vi "vipm_OpenVIPM.vi"(8 "error in (no error)":errorcluster, 11 "CommandLine":string[](array[string])) -> (0 "error out":errorcluster, 2 "test details":string, 3 "output to action":string)   [LabVIEW 2014]
uses:
  _lvcicd/_lvcicd_support_2014.lvlib
  <vilib>/JKI/VIPM API/VIPM API_vipm_api.lvlib
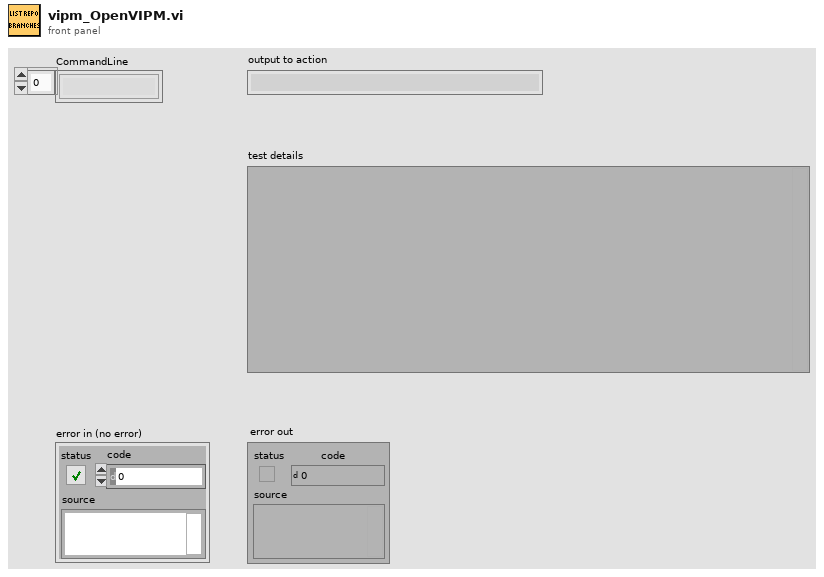
[diagram p1: front panel]
types:
  T1 = typedef "VIPM API_vipm_api.lvlib/LabVIEW Target Info Cluster_vipm_api.ctl" = cluster{"Version":string, "Connection Tested":bool, "Disabled":bool}
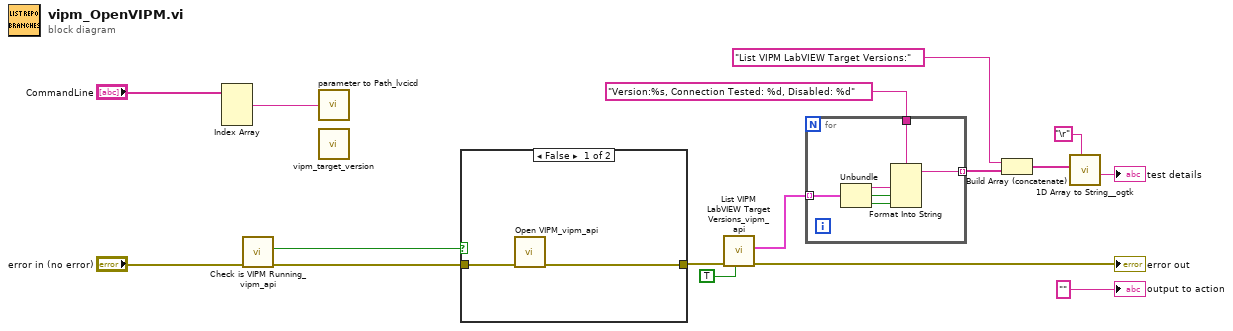
[diagram p0: block diagram]
diagram:
  n1 = Index Array(array="CommandLine") -> (element #1=w15:string)  [unwired: 3 in, 2 out]
  n2 = call <vilib>:"Check is VIPM Running_vipm_api.vi"("error in (no error)"="error in (no error)") -> ("error out"=w14:errorcluster, "is Running"=w11:bool)  [unwired: 9 in]
  n3 = call "parameter to Path_lvcicd.vi"("String"=w15) -> ()  [unwired: 1 out]
  n4 = call "vipm_target_version.vi"() -> ()  [unwired: 11 in, 1 out]
  n5 = case shown="False" w11 {
    tunnel: w14 -> [w18 w19]
    tunnel: [w17 w19] -> w10
    frame False {
      n6 = call <vilib>:"Open VIPM_vipm_api.vi"("error in (no error)"=w18) -> ("error out"=w17:errorcluster)  [unwired: 10 in]
    }
    frame True {
    }
  }
  n7 = call <vilib>:"List VIPM LabVIEW Target Versions_vipm_api.vi"("List Invalid Targets? (F)"=TRUE, "error in (no error)"=w10) -> ("error out"=→"error out":errorcluster, "LabVIEW Target Info"=w7:T1[])  [unwired: 8 in]
  n8 = for {
    tunnel: w7 -> [w25] mode=indexing
    tunnel: "Version:%s, Connection Tested: %d, Disabled: %d" ("format string") -> [w21]
    tunnel: [w20] -> w5 mode=indexing
    n9 = Unbundle(w25) -> ("Version"=w24:string, "Connection Tested"=w23:bool, "Disabled"=w22:bool)
    n10 = Format Into String(format string=w21, w24, w23, w22) -> (resulting string=w20:string)  [unwired: 2 in, 1 out]
  }
  n11 = Build Array (concatenate)("List VIPM LabVIEW Target Versions:" ("format string"), w5) -> (w2:string[])
  n12 = call <userlib>:"1D Array to String__ogtk.vi"("delimiter (Tab)"="\r", "Array of Strings"=w2) -> ("delimited string"=→"test details":string)  [unwired: 9 in]
  "output to action" <- "" ("test details")
